vi "Menu_Named Bundler.vi"(11 "Affected Items Out":T1) -> (3 "Menu Items To Add":T2(array[cluster]))   [LabVIEW 2023]
uses:
  top/BundleMagic.ctl
  controls/action enum.ctl
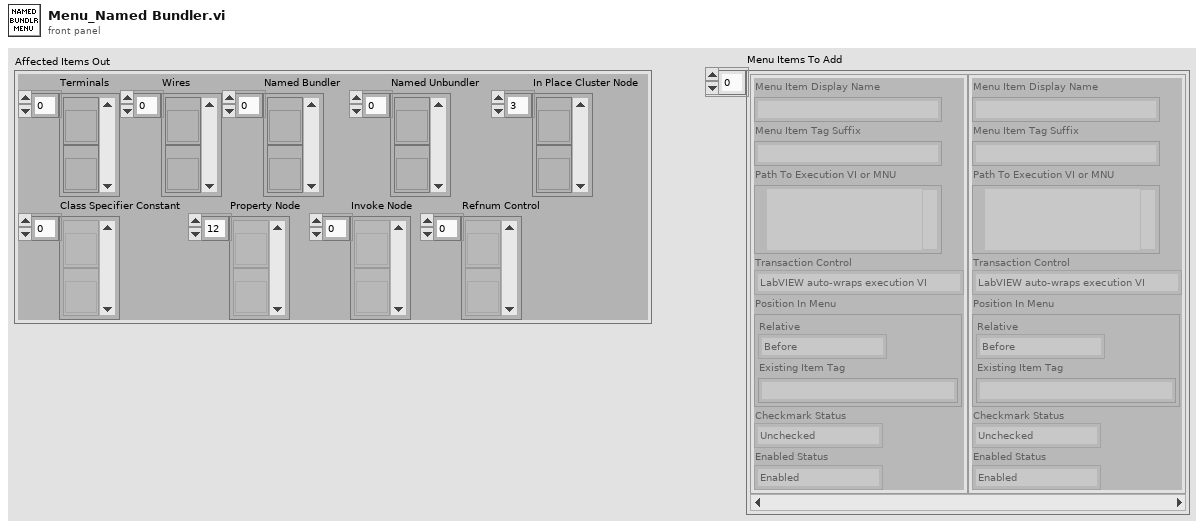
[diagram p1: front panel]
types:
  T1 = typedef "BundleMagic.ctl" = cluster{"Terminals":refnum<vi>[], "Wires":refnum<vi>[], "Named Bundler":refnum<vi>[], "Named Unbundler":refnum<vi>[], "In Place Cluster Node":refnum<vi>[], "Class Specifier Constant":refnum<vi>[], "Property Node":refnum<vi>[], "Invoke Node":refnum<vi>[], "Refnum Control":refnum<vi>[]}
  T2 = cluster{"Menu Item Display Name":string, "Menu Item Tag Suffix":string, "Path To Execution VI or MNU":path, "Transaction Control":enum8{"LabVIEW auto-wraps execution VI", "Execution VI will define if needed"}, "Position In Menu":cluster{"Relative":enum8{"Before", "Instead of", "After", "Into Submenu"}, "Existing Item Tag":string}, "Checkmark Status":enum8{"Unchecked", "Checked"}, "Enabled Status":enum8{"Enabled", "Disabled"}}[]
  T3 = typedef "action enum.ctl" = enum16{"[NONE]", "APP_SEPARATOR", "Wire Bundle", "Wire Unbundle", "Terminal Unbundle", "Terminal Bundle", "Bundler Move Up", "Bundler Move Down", "Bundler Insert", "Bundler Remove", "Bundler Remove Unwired", "Bundler Rearrange", "In Place Insert", "In Place Remove", "In Place Remove Unwired", "In Place Rearrange", "Wire Properties", "Wire Method", "Terminal Properties", "Terminal Method", "Property Move Up", "Property Move Down", "Properties Insert", "Properties Remove", "Properties Remove Unwired", "Properties Rearrange", "Method Change", "Class For Constant", "Class For Control", "Class For Node", "Class Name to Clipboard"}
  T4 = cluster{"Relative":enum8{"Before", "Instead of", "After", "Into Submenu"}, "Existing Item Tag":string}[]
  T5 = cluster{"Menu Item Display Name":string, "Menu Item Tag Suffix":string, "Path To Execution VI or MNU":path, "Transaction Control":enum8{"LabVIEW auto-wraps execution VI", "Execution VI will define if needed"}, "Position In Menu":cluster{"Relative":enum8{"Before", "Instead of", "After", "Into Submenu"}, "Existing Item Tag":string}, "Checkmark Status":enum8{"Unchecked", "Checked"}, "Enabled Status":enum8{"Enabled", "Disabled"}}
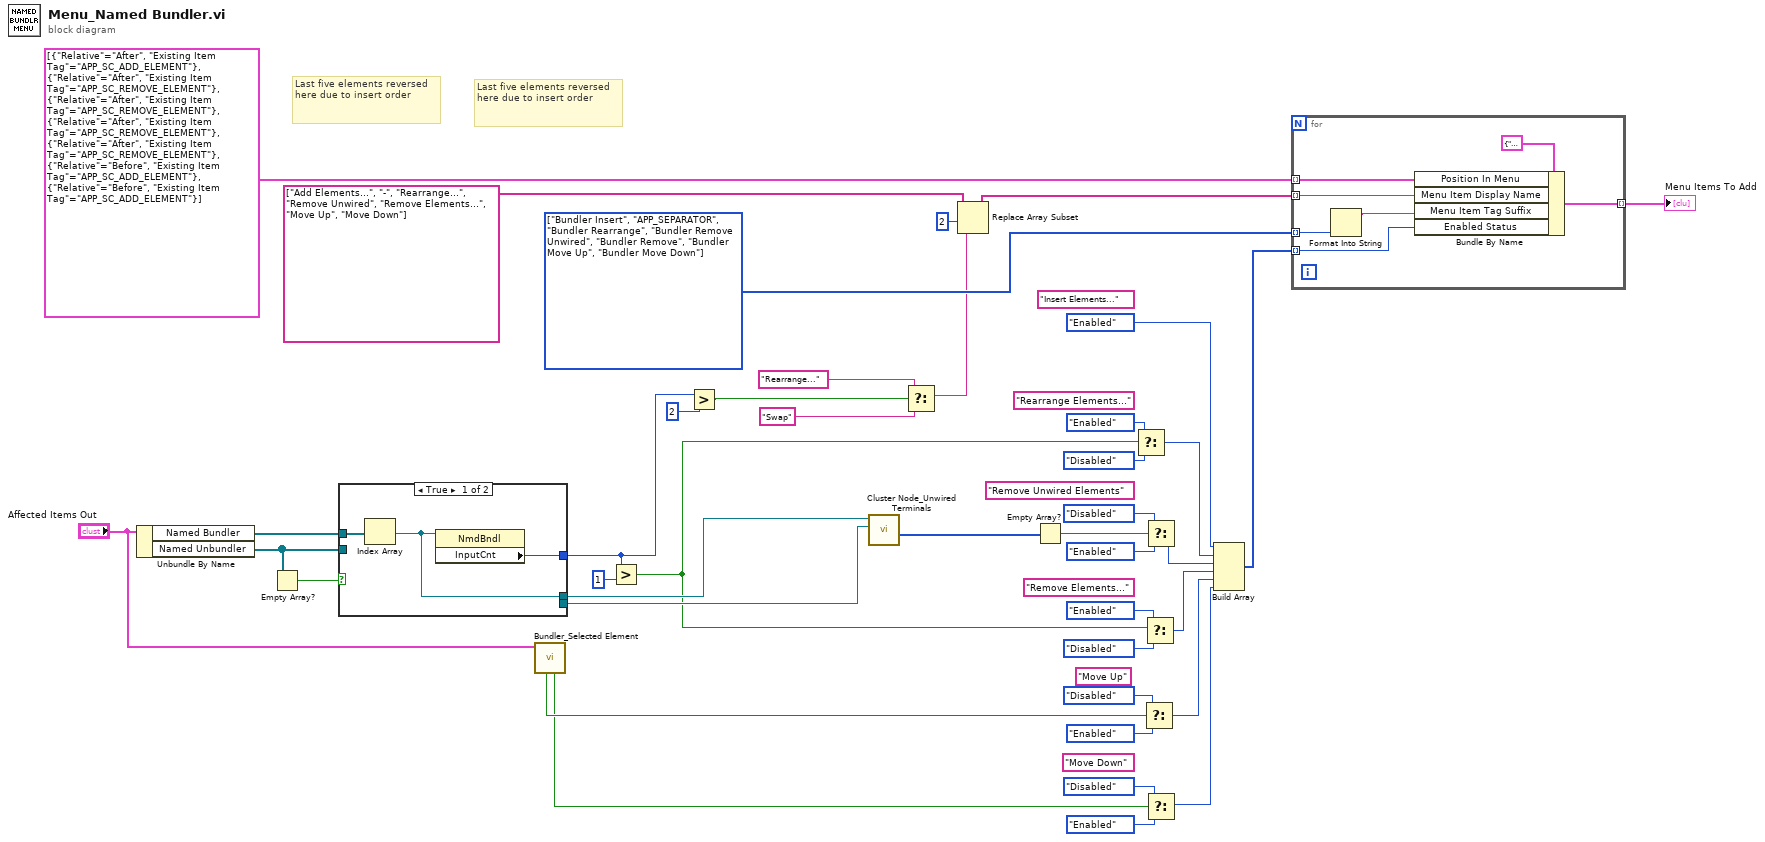
[diagram p0: block diagram]
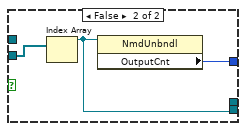
[diagram p2: hidden frame]
diagram:
  (unwired) "Move Up" ("Menu Item Display Name")
  (unwired) "Move Down" ("Menu Item Display Name")
  (unwired) "Remove Elements..." ("Menu Item Display Name")
  (unwired) "Remove Unwired Elements" ("Menu Item Display Name")
  (unwired) "Rearrange Elements..." ("Menu Item Display Name")
  (unwired) "Insert Elements..." ("Menu Item Display Name")
  w39 = T3[] [enum."Bundler Insert", enum."APP_SEPARATOR", enum."Bundler Rearrange", enum."Bundler Remove Unwired", enum."Bundler Remove", enum."Bundler Move Up", enum."Bundler Move Down"] items=["[NONE]", "APP_SEPARATOR", "Wire Bundle", "Wire Unbundle", "Terminal Unbundle", "Terminal Bundle", "Bundler Move Up", "Bundler Move Down", "Bundler Insert", "Bundler Remove", "Bundler Remove Unwired", "Bundler Rearrange", "In Place Insert", "In Place Remove", "In Place Remove Unwired", "In Place Rearrange", "Wire Properties", "Wire Method", "Terminal Properties", "Terminal Method", "Property Move Up", "Property Move Down", "Properties Insert", "Properties Remove", "Properties Remove Unwired", "Properties Rearrange", "Method Change", "Class For Constant", "Class For Control", "Class For Node", "Class Name to Clipboard"] ("Enabled Status")
  # "Last five elements reversed here due to insert order"
  # "Last five elements reversed here due to insert order"
  n1 = Unbundle By Name("Affected Items Out") -> ("Named Bundler"=w36:refnum<vi>[], "Named Unbundler"=w35:refnum<vi>[])
  n2 = Empty Array?(array=w35) -> (empty?=w37:bool)
  n3 = case shown="True" w37 {
    tunnel: [w44 w47] -> w9
    tunnel: w36 -> [w43 _]
    tunnel: w35 -> [_ w46]
    tunnel: [w42 _] -> w30
    tunnel: [_ w45] -> w29
    frame True {
      n4 = Index Array(array=w43) -> (element=w42:refnum<vi>)  [unwired: 1 in]
      n5 = property class="NmdBndl"(reference=w42) -> ("InputCnt"=w44:i32)  [unwired: 1 in, 2 out]
    }
    frame False {
      n6 = Index Array(array=w46) -> (element=w45:refnum<vi>)  [unwired: 1 in]
      n7 = property class="NmdUnbndl"(reference=w45) -> ("OutputCnt"=w47:i32)  [unwired: 1 in, 2 out]
    }
  }
  n8 = call "Bundler_Selected Element.vi"("Affected Items"="Affected Items Out") -> ("last element"=w3:bool, "first element"=w4:bool)  [unwired: 4 in, 5 out]
  n9 = Greater?(x=w9, y=1) -> (0:w12:bool)
  n10 = Greater?(x=w9, y=2) -> (0:w7:bool)
  n11 = call "Cluster Node_Unwired Terminals.vi"("Named Unbundler Ref"=w29, "Named Bundler Ref"=w30) -> ("Unwired Indices For Removal"=w32:i32[])  [unwired: 7 in, 2 out]
  n12 = Select(t="Rearrange..." ("Menu Item Display Name"), s=w7, f="Swap" ("Menu Item Display Name")) -> (s? t:f=w5:string)
  n13 = Replace Array Subset(array=string[] ["Add Elements...", "-", "Rearrange...", "Remove Unwired", "Remove Elements...", "Move Up", "Move Down"], new element=w5, index=2) -> (w1:string[])
  n14 = Empty Array?(array=w32) -> (empty?=w31:bool)
  n15 = Select(t=enum8{"Enabled", "Disabled"}."Enabled" ("Enabled Status"), s=w12, f=enum8{"Enabled", "Disabled"}."Disabled" ("Enabled Status")) -> (s? t:f=w24:enum8{"Enabled", "Disabled"})
  n16 = Select(t=enum8{"Enabled", "Disabled"}."Disabled" ("Enabled Status"), s=w4, f=enum8{"Enabled", "Disabled"}."Enabled" ("Enabled Status")) -> (s? t:f=w15:enum8{"Enabled", "Disabled"})
  n17 = Select(t=enum8{"Enabled", "Disabled"}."Enabled" ("Enabled Status"), s=w12, f=enum8{"Enabled", "Disabled"}."Disabled" ("Enabled Status")) -> (s? t:f=w20:enum8{"Enabled", "Disabled"})
  n18 = Select(t=enum8{"Enabled", "Disabled"}."Disabled" ("Enabled Status"), s=w31, f=enum8{"Enabled", "Disabled"}."Enabled" ("Enabled Status")) -> (s? t:f=w23:enum8{"Enabled", "Disabled"})
  n19 = Select(t=enum8{"Enabled", "Disabled"}."Disabled" ("Enabled Status"), s=w3, f=enum8{"Enabled", "Disabled"}."Enabled" ("Enabled Status")) -> (s? t:f=w14:enum8{"Enabled", "Disabled"})
  n20 = Build Array(enum8{"Enabled", "Disabled"}."Enabled" ("Enabled Status"), w24, w23, w20, w15, w14) -> (w27:enum8{"Enabled", "Disabled"}[])
  n21 = for {
    tunnel: [w54] -> w40 mode=indexing
    tunnel: w1 -> [w53] mode=indexing
    tunnel: T4 [{"Relative"=enum."After", "Existing Item Tag"="APP_SC_ADD_ELEMENT"}, {"Relative"=enum."After", "Existing Item Tag"="APP_SC_REMOVE_ELEMENT"}, {"Relative"=enum."After", "Existing Item Tag"="APP_SC_REMOVE_ELEMENT"}, {"Relative"=enum."After", "Existing Item Tag"="APP_SC_REMOVE_ELEMENT"}, {"Relative"=enum."After", "Existing Item Tag"="APP_SC_REMOVE_ELEMENT"}, {"Relative"=enum."Before", "Existing Item Tag"="APP_SC_ADD_ELEMENT"}, {"Relative"=enum."Before", "Existing Item Tag"="APP_SC_ADD_ELEMENT"}] -> [w51] mode=indexing
    tunnel: w27 -> [w50] mode=indexing
    tunnel: w39 -> [w48] mode=indexing
    n22 = Format Into String(w48) -> (resulting string=w49:string)  [unwired: 3 in, 1 out]
    n23 = Bundle By Name(cluster=T5 {"Menu Item Display Name"="", "Menu Item Tag Suffix"="", "Path To Execution VI or MNU"=path "", "Transaction Control"=enum."LabVIEW auto-wraps execution VI", "Position In Menu"={"Relative"=enum."Before", "Existing Item Tag"=""}, "Checkmark Status"=enum."Unchecked", "Enabled Status"=enum."Enabled"} ("Cluster"), "Position In Menu"=w51, "Menu Item Display Name"=w53, "Menu Item Tag Suffix"=w49, "Enabled Status"=w50) -> (w54:T5)
  }
  "Menu Items To Add" <- w40
